vi "Update.vi"(8 "error in (no error)":errorcluster, 10 "Message in":refnum<class "UpdateMessage.lvclass">, 11 "RSA in":refnum<class "RSA.lvclass">) -> (0 "error out":errorcluster, 3 "RSA out":refnum<class "RSA.lvclass">)   [LabVIEW 2012, in "RSA.lvclass"]
doc: "The update method processes the command 'update'. \n\nThe command 'update' is used for receiving new values to be set to the private data of the class. This could be seen as a public set method for setting new parameters to the private class data."
uses:
  RSA.lvclass
  <vilib>/Distrio/Murmex/UpdateMessage/UpdateMessage.lvclass
  RSA.lvclass/RSA.ctl
  starting shape.ctl
  <vilib>/Distrio/Murmex/Murmex/Murmex.lvclass
panel:
  # "This method is called when the UPDATE\ntrigger is sent. \n\nOverride this method when your component needs to\nrespond to this trigger. \n\nCall parent for proper implementation"
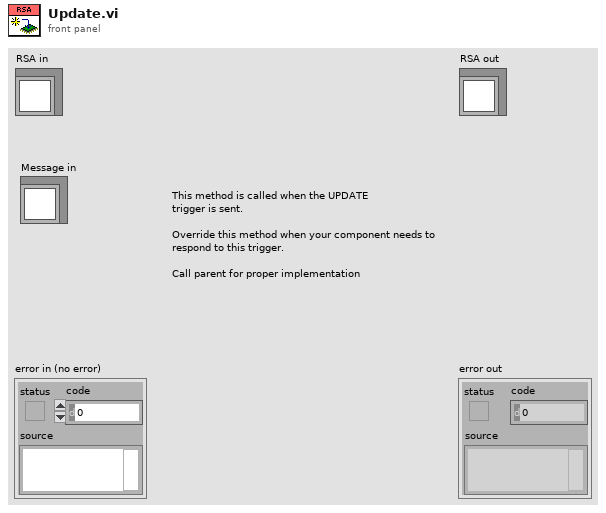
[diagram p1: front panel]
types:
  T1 = typedef "RSA.lvclass/starting shape.ctl" = enum16{"Load shape", "Midrange"}
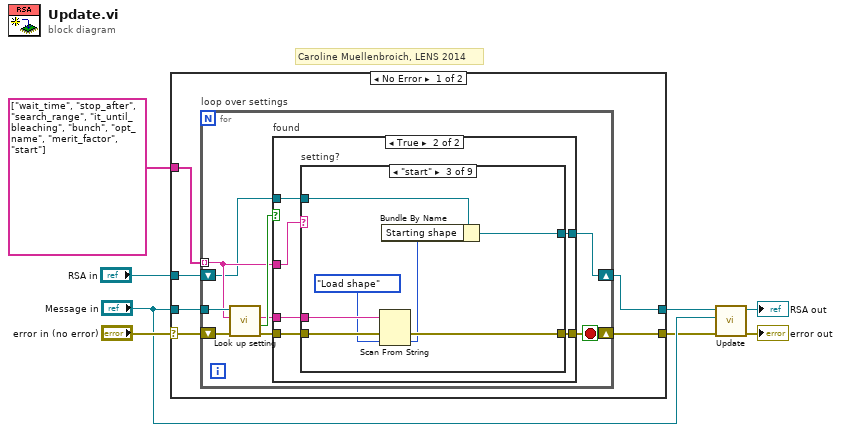
[diagram p0: block diagram]
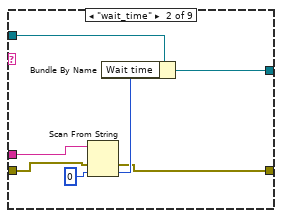
[diagram p4: hidden frame]
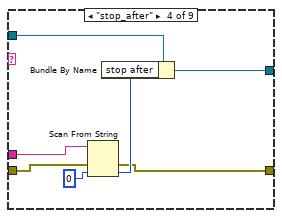
[diagram p5: hidden frame]
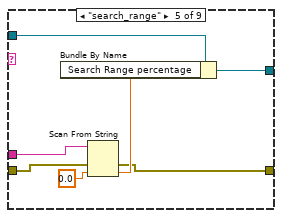
[diagram p6: hidden frame]
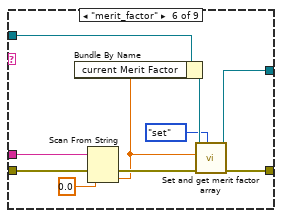
[diagram p7: hidden frame]
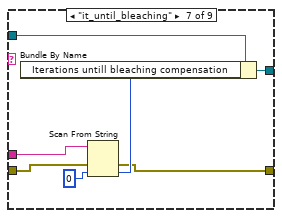
[diagram p8: hidden frame]
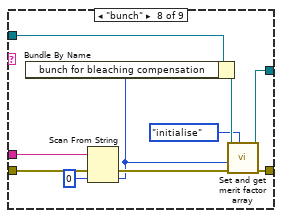
[diagram p9: hidden frame]
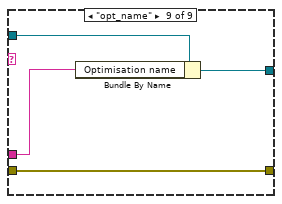
[diagram p10: hidden frame]
diagram:
  # "Caroline Muellenbroich, LENS 2014"
  n1 = case shown="No Error" "error in (no error)" {
    selector: "error in (no error)" -> [w14 w94]
    tunnel: "Message in" -> [w13 _]
    tunnel: string[] ["wait_time", "stop_after", "search_range", "it_until_bleaching", "bunch", "opt_name", "merit_factor", "start"] ("key chains") -> [w12 _]
    tunnel: "RSA in" -> [w11 w93]
    tunnel: [w10 w94] -> w3
    tunnel: [w9 w93] -> w2
    frame No Error {
      n2 = for "loop over settings" {
        shift-right: [w15] -> w10
        shift-left: w14 -> [w23]
        tunnel: w13 -> [w22]
        tunnel: w12 -> [w19] mode=indexing
        shift-right: [w18] -> w9
        shift-left: w11 -> [w17]
        stop <- w15 stop-if-true
        n3 = call <vilib>:"Look up setting.vi"("error in (no error)"=w23, "tag name"=w19, "UpdateMessage in"=w22) -> ("error out"=w16:errorcluster, "found?"=w21:bool, "value"=w20:string)  [unwired: 5 in, 1 out]
        n4 = case "found" shown="True" w21 {
          tunnel: w20 -> [_ w30]
          tunnel: w19 -> [_ w31]
          tunnel: [w24 w29] -> w18
          tunnel: w17 -> [w24 w28]
          tunnel: w16 -> [w25 w27]
          tunnel: [w25 w26] -> w15
          frame False {
          }
          frame True {
            n5 = case "setting?" shown="\"start\"" w31 {
              tunnel: w30 -> [_ w40 w47 w54 w61 w71 w78 w88 w90]
              tunnel: [w33 w39 w46 w53 w60 w66 w77 w83 w92] -> w29
              tunnel: w28 -> [w33 w38 w45 w52 w59 w70 w76 w87 w91]
              tunnel: [w32 w34 w43 w48 w55 w64 w72 w81 w89] -> w26
              tunnel: w27 -> [w32 w35 w44 w49 w56 w68 w73 w85 w89]
              frame "False", Default {
              }
              frame "wait_time" {
                n6 = Scan From String(input string=w40, error in=w35, default 1=u32 0 ("Settings Cluster.Wait time")) -> (error out=w34:errorcluster, output 1=w36:u32)  [unwired: 2 in, 2 out]
                n7 = Bundle By Name(cluster=w38, "Wait time"=w36) -> (w39:refnum<class "RSA.lvclass">)
              }
              frame "start" {
                n8 = Scan From String(input string=w47, error in=w44, default 1=starting_shape."Load shape" ("Settings Cluster.Starting shape")) -> (error out=w43:errorcluster, output 1=w41:T1)  [unwired: 2 in, 2 out]
                n9 = Bundle By Name(cluster=w45, "Starting shape"=w41) -> (w46:refnum<class "RSA.lvclass">)
              }
              frame "stop_after" {
                n10 = Scan From String(input string=w54, error in=w49, default 1=0 ("Settings Cluster.stop after")) -> (error out=w48:errorcluster, output 1=w51:i32)  [unwired: 2 in, 2 out]
                n11 = Bundle By Name(cluster=w52, "stop after"=w51) -> (w53:refnum<class "RSA.lvclass">)
              }
              frame "search_range" {
                n12 = Scan From String(input string=w61, error in=w56, default 1=0.0 ("Settings Cluster.stop after")) -> (error out=w55:errorcluster, output 1=w58:dbl)  [unwired: 2 in, 2 out]
                n13 = Bundle By Name(cluster=w59, "Search Range percentage"=w58) -> (w60:refnum<class "RSA.lvclass">)
              }
              frame "merit_factor" {
                n14 = Scan From String(input string=w71, error in=w68, default 1=0.0 ("Settings Cluster.stop after")) -> (error out=w65:errorcluster, output 1=w63:dbl)  [unwired: 2 in, 2 out]
                n15 = Bundle By Name(cluster=w70, "current Merit Factor"=w63) -> (w67:refnum<class "RSA.lvclass">)
                n16 = call "Set and get merit factor array.vi"("action"=enum16{"set", "get", "initialise"}."set", "error in (no error)"=w65, "merit factor"=w63, "RSA in"=w67) -> ("error out"=w64:errorcluster, "RSA out"=w66:refnum<class "RSA.lvclass">)  [unwired: 4 in, 2 out]
              }
              frame "it_until_bleaching" {
                n17 = Scan From String(input string=w78, error in=w73, default 1=0 ("Settings Cluster.stop after")) -> (error out=w72:errorcluster, output 1=w75:i32)  [unwired: 2 in, 2 out]
                n18 = Bundle By Name(cluster=w76, "Iterations untill bleaching compensation"=w75) -> (w77:refnum<class "RSA.lvclass">)
              }
              frame "bunch" {
                n19 = Scan From String(input string=w88, error in=w85, default 1=0 ("Settings Cluster.stop after")) -> (error out=w82:errorcluster, output 1=w79:i32)  [unwired: 2 in, 2 out]
                n20 = Bundle By Name(cluster=w87, "bunch for bleaching compensation"=w79) -> (w84:refnum<class "RSA.lvclass">)
                n21 = call "Set and get merit factor array.vi"("action"=enum16{"set", "get", "initialise"}."initialise", "error in (no error)"=w82, "array size"=w79, "RSA in"=w84) -> ("error out"=w81:errorcluster, "RSA out"=w83:refnum<class "RSA.lvclass">)  [unwired: 4 in, 2 out]
              }
              frame "opt_name" {
                n22 = Bundle By Name(cluster=w91, "Optimisation name"=w90) -> (w92:refnum<class "RSA.lvclass">)
              }
            }
          }
        }
      }
    }
    frame Error {
    }
  }
  n23 = call-parent "Update.vi"("error in (no error)"=w3, "Message in"="Message in", "Murmex in"=w2) -> ("error out"=→"error out":errorcluster, "Murmex out"=→"RSA out":refnum<class "RSA.lvclass">)  [unwired: 7 in]
